vi "NE-500 FGV.vi"(7 "Function":T2(ring), 8 "error in":errorcluster, 10 "Setting":T1, 11 "VISA resource":refnum<visa-resource-name>) -> (0 "error out":errorcluster, 3 "Read String":string)   [LabVIEW 2019, in "NE-500.lvlib"]
uses:
  NE-500.lvlib
  <vilib>/Instr/_visa.llb/VISA Configure Serial Port (Instr).vi
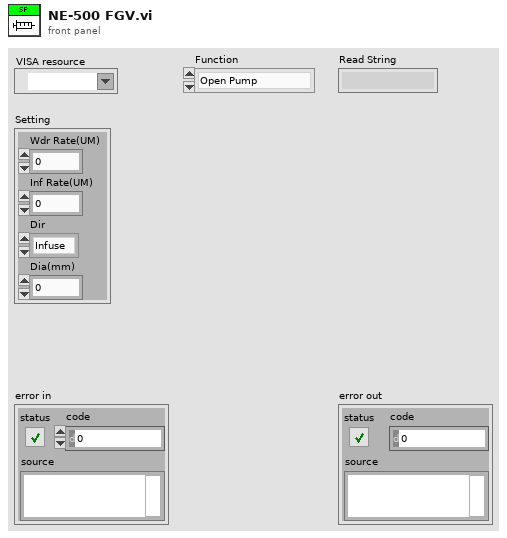
[diagram p1: front panel]
types:
  T1 = cluster{"Wdr Rate(UM)":dbl, "Inf Rate(UM)":dbl, "Dir":enum16{"Infuse", "Withdraw"}, "Dia(mm)":dbl}
  T2 = enum16{"Open Pump", "Read", "Set", "Run", "Stop", "Close Pump"}
  T3 = cluster{"Syringe Pump Setting":cluster{"Wdr Rate(UM)":dbl, "Inf Rate(UM)":dbl, "Dir":enum16{"Infuse", "Withdraw"}, "Dia(mm)":dbl}, "On/Off":bool, "VISA resource":refnum<visa-resource-name>, "Read String":string}
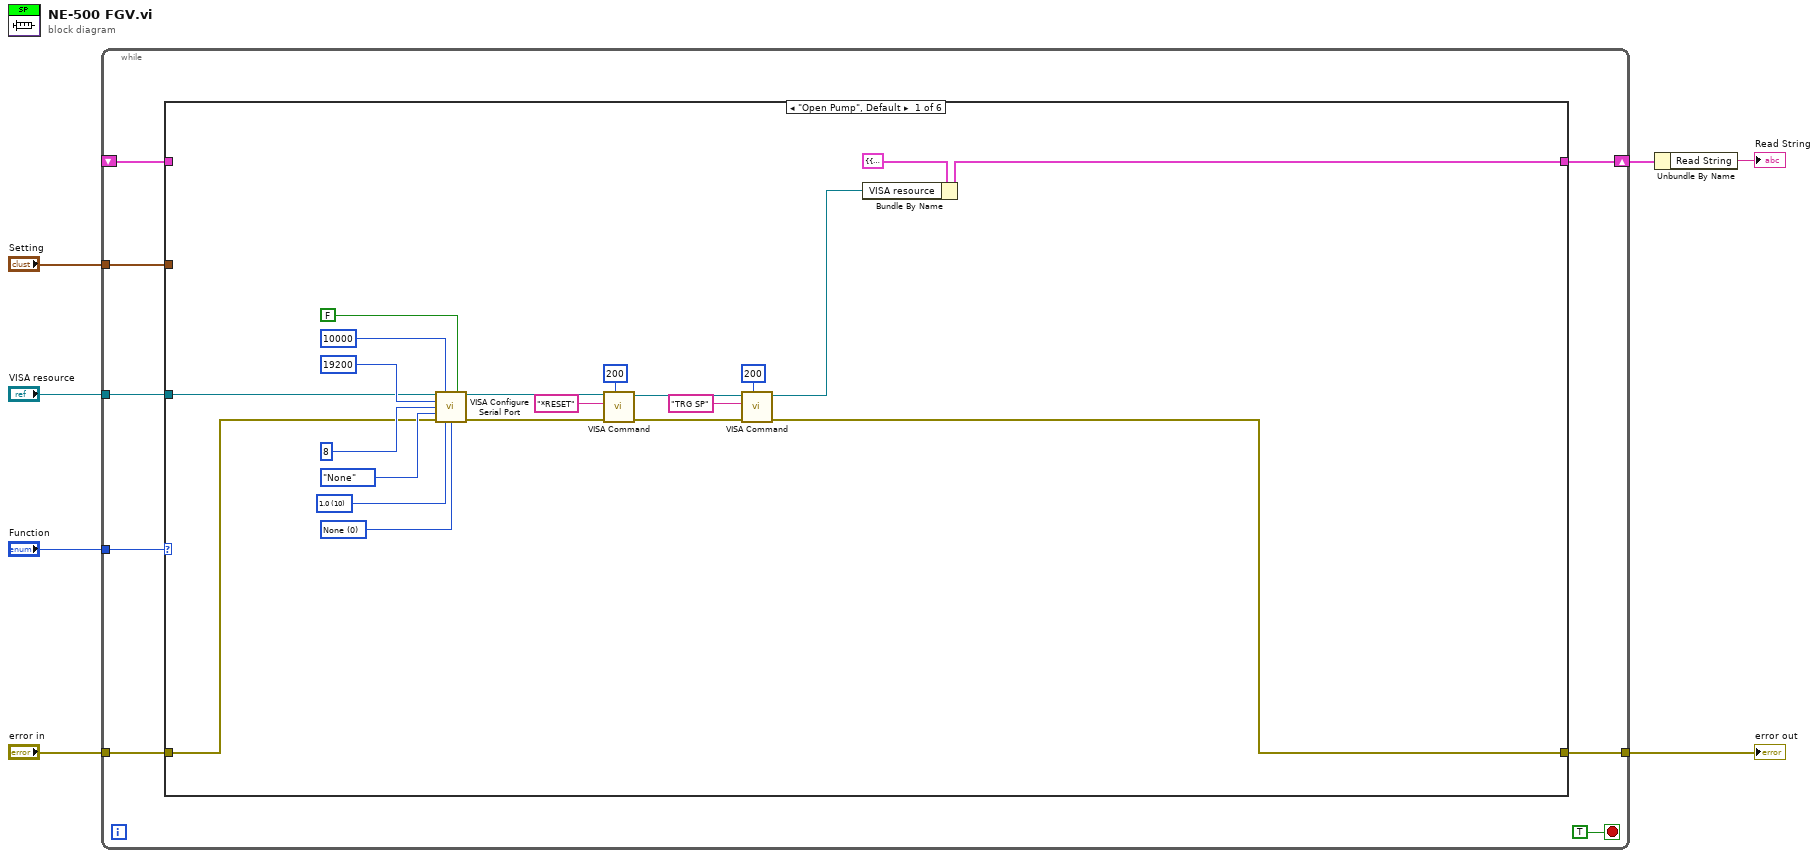
[diagram p0: block diagram]
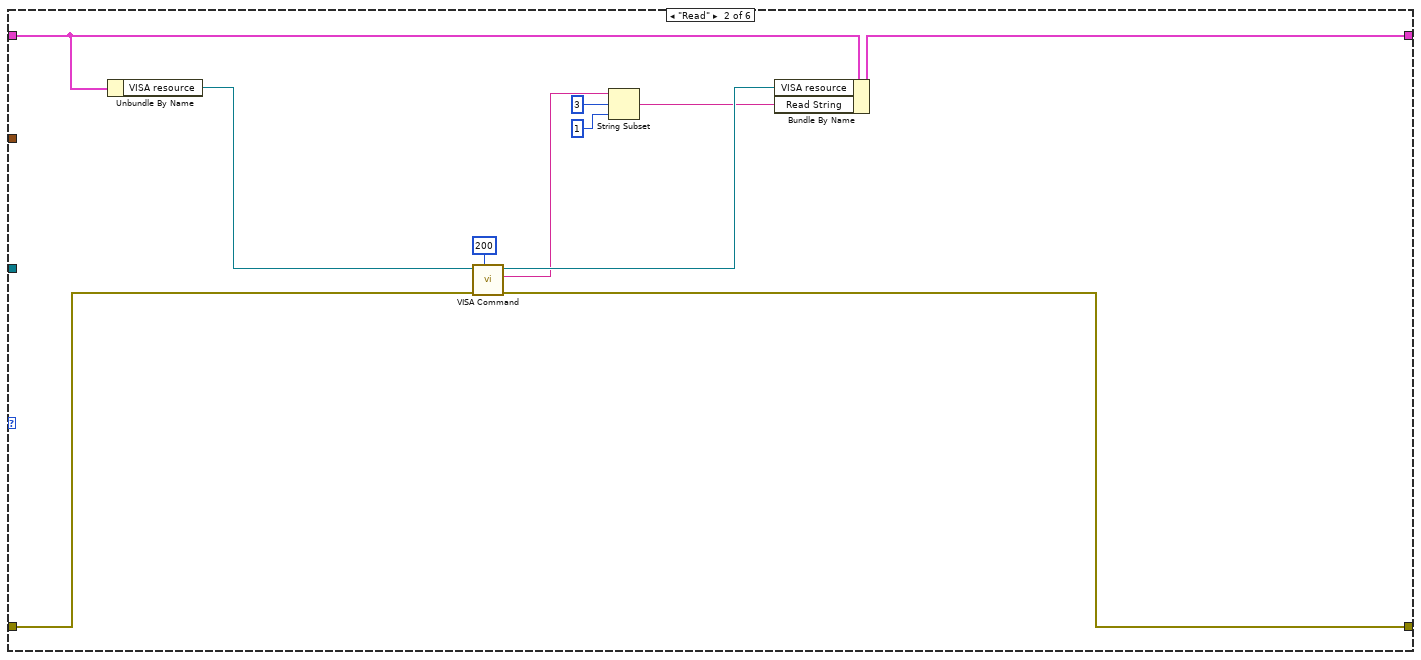
[diagram p2: hidden frame]
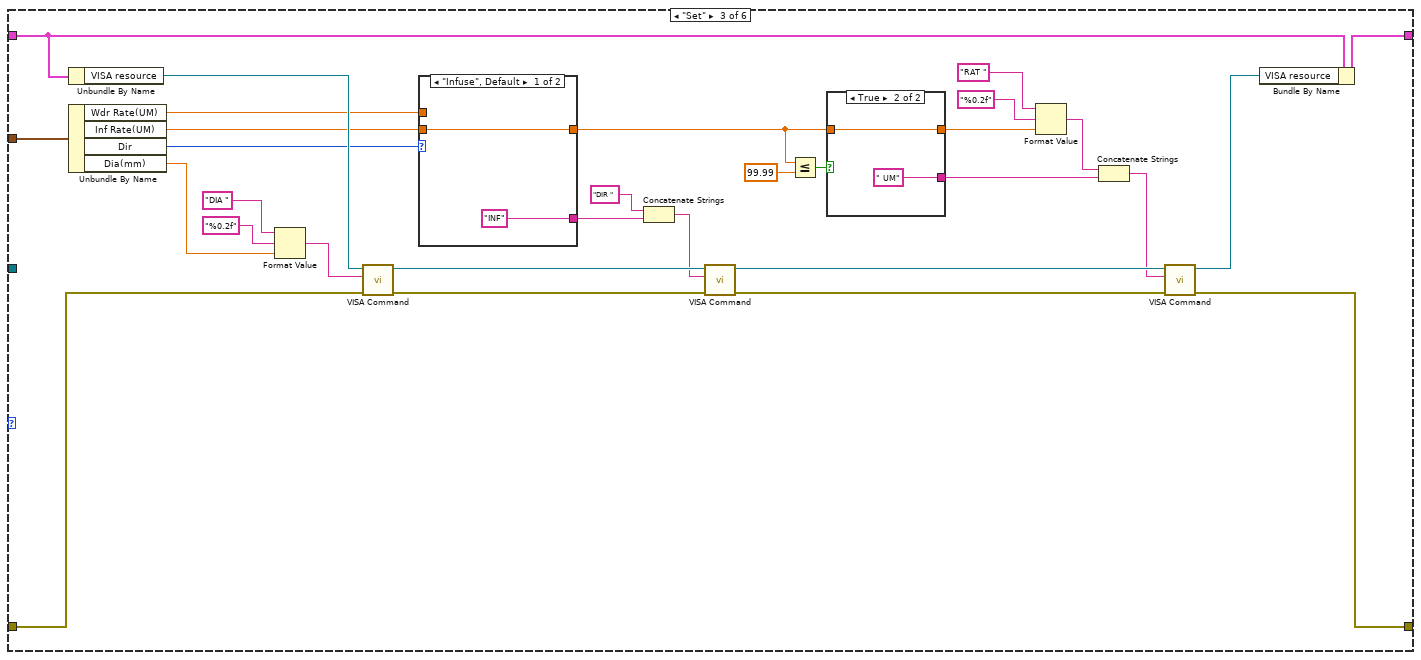
[diagram p3: hidden frame]
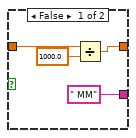
[diagram p4: hidden frame]
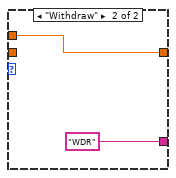
[diagram p5: hidden frame]
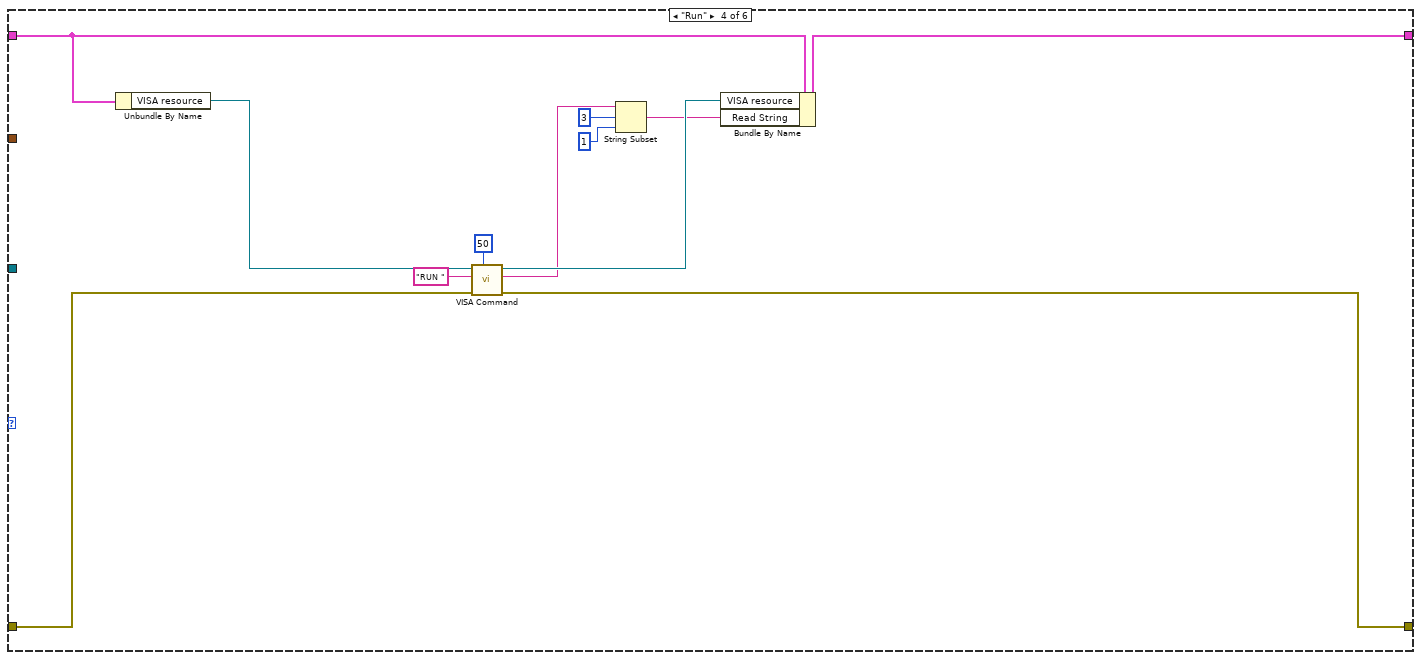
[diagram p6: hidden frame]
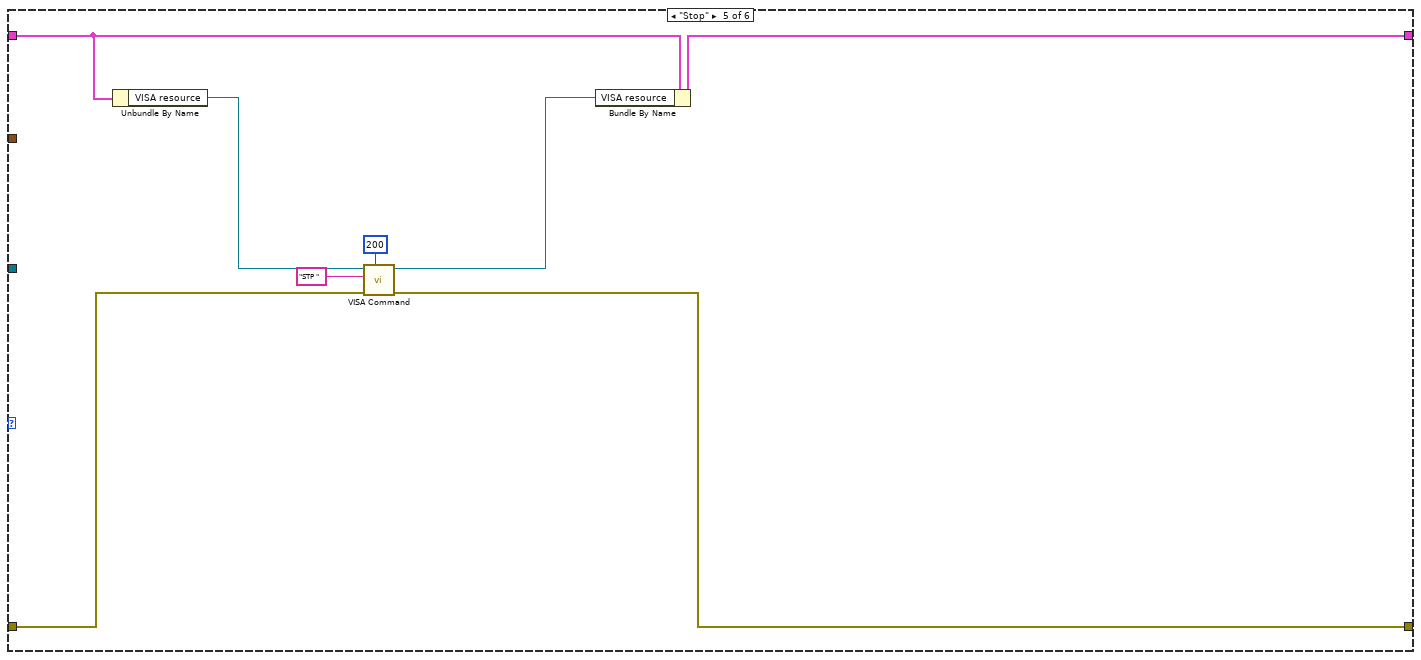
[diagram p7: hidden frame]
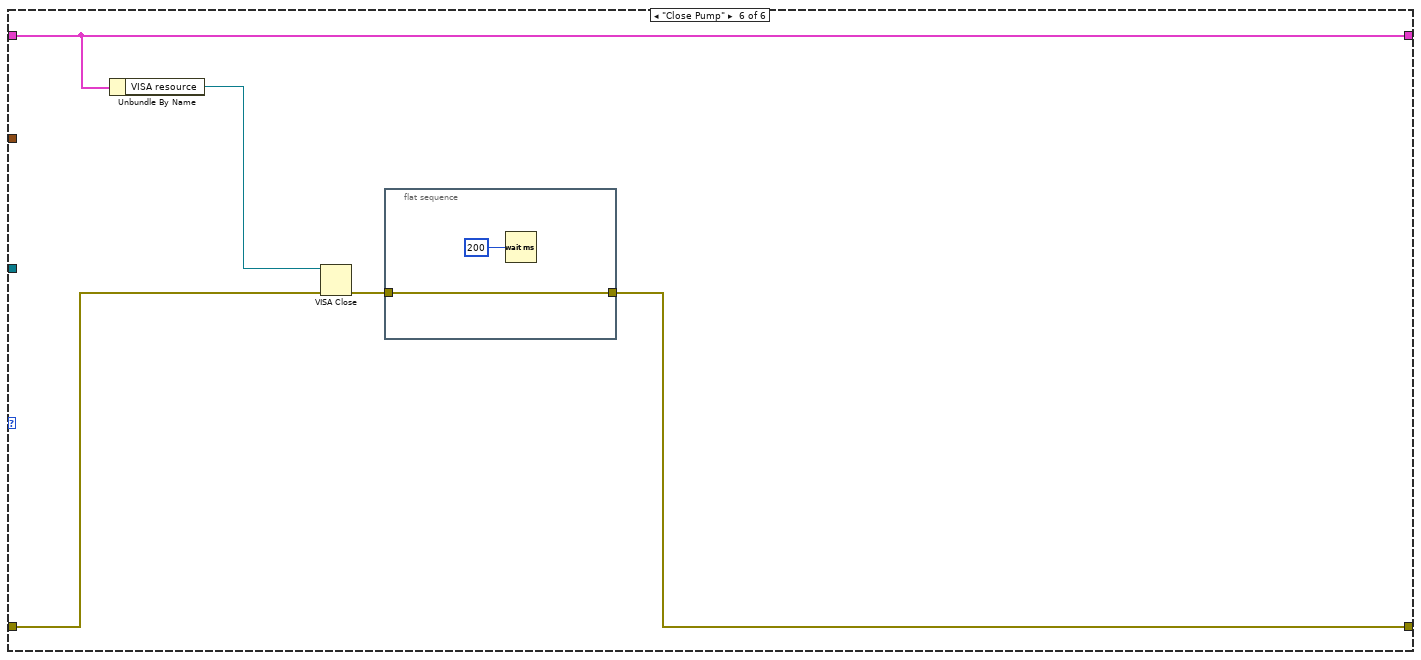
[diagram p8: hidden frame]
diagram:
  n1 = while {
    tunnel: "Function" -> [w14]
    shift-right: [w12] -> w2
    shift-left: _ -> [w13]
    tunnel: "VISA resource" -> [w11]
    tunnel: "error in" -> [w10]
    tunnel: [w9] -> w4
    tunnel: "Setting" -> [w8]
    stop <- TRUE stop-if-true
    n2 = case shown="\"Open Pump\", Default" w14 {
      tunnel: w13 -> [_ w45 w65 w97 w105 w111]
      tunnel: [w27 w44 w57 w93 w101 w111] -> w12
      tunnel: w11 -> [w28 _ _ _ _ _]
      tunnel: w10 -> [w29 w47 w71 w99 w107 w112]
      tunnel: [w18 w46 w68 w98 w102 w108] -> w9
      tunnel: w8 -> [_ _ w67 _ _ _]
      frame "Open Pump", Default {
        w33 = u16 0 items=["None"=0, "XON/XOFF"=1, "RTS/CTS"=2, "DTR/DSR"=4] ("flow control")
        w32 = u16 10 items=["1.0"=10, "1.5"=15, "2.0"=20] ("stop bits")
        n3 = call-poly "VISA Configure Serial Port"("VISA resource name"=w28, "timeout (10sec)"=u32 10000, "Enable Termination\nChar (T)"=FALSE ("Enable Termination Char (T)"), "baud rate (9600)"=u32 19200 ("baud rate"), "data bits (8)"=u16 8 ("data bits"), "parity (0:none)"=enum16{"None", "Odd", "Even", "Mark", "Space"}."None", "error in (no error)"=w29, "stop bits (10: 1 bit)"=w32, "flow control (0:none)"=w33) -> ("VISA resource name out"=w25:refnum<visa-resource-name>, "error out"=w26:errorcluster)  [unwired: 5 out]
        n4 = call "VISA Command.vi"("Wait (ms)"=u32 200, "error in (no error)"=w26, "Command"="*RESET" ("CMD string"), "VISA resource name"=w25) -> ("error out"=w24:errorcluster, "VISA resource name out"=w21:refnum<visa-resource-name>)  [unwired: 5 in, 1 out]
        n5 = call "VISA Command.vi"("Wait (ms)"=u32 200, "error in (no error)"=w24, "Command"="TRG SP" ("CMD string"), "VISA resource name"=w21) -> ("error out"=w18:errorcluster, "VISA resource name out"=w17:refnum<visa-resource-name>)  [unwired: 5 in, 1 out]
        n6 = Bundle By Name(cluster=T3 {"Syringe Pump Setting"={"Wdr Rate(UM)"=0.0, "Inf Rate(UM)"=0.0, "Dir"=enum."Infuse", "Dia(mm)"=0.0}, "On/Off"=FALSE, "VISA resource"="", "Read String"=""}, "VISA resource"=w17) -> (w27:T3)
      }
      frame "Read" {
        n7 = Unbundle By Name(w45) -> ("VISA resource"=w43:refnum<visa-resource-name>)
        n8 = call "VISA Command.vi"("Wait (ms)"=u32 200, "error in (no error)"=w47, "VISA resource name"=w43) -> ("error out"=w46:errorcluster, "read buffer"=w38:string, "VISA resource name out"=w42:refnum<visa-resource-name>)  [unwired: 6 in]
        n9 = String Subset(string=w38, offset (0)=3, length (rest)=1 ("length (rest)")) -> (substring=w37:string)
        n10 = Bundle By Name(cluster=w45, "VISA resource"=w42, "Read String"=w37) -> (w44:T3)
      }
      frame "Set" {
        n11 = Unbundle By Name(w65) -> ("VISA resource"=w64:refnum<visa-resource-name>)
        n12 = Unbundle By Name(w67) -> ("Wdr Rate(UM)"=w61:dbl, "Inf Rate(UM)"=w60:dbl, "Dir"=w62:enum16{"Infuse", "Withdraw"}, "Dia(mm)"=w63:dbl)
        n13 = Format Value(string ("")="DIA ", format string="%0.2f", value (0)=w63) -> (output string=w66:string)
        n14 = call "VISA Command.vi"("error in (no error)"=w71, "Command"=w66, "VISA resource name"=w64) -> ("error out"=w70:errorcluster, "VISA resource name out"=w59:refnum<visa-resource-name>)  [unwired: 6 in, 1 out]
        n15 = case shown="\"Infuse\", Default" w62 {
          tunnel: w61 -> [_ w86]
          tunnel: w60 -> [w84 _]
          tunnel: ["INF" "WDR"] -> w55
          tunnel: [w84 w86] -> w51
          frame "Infuse", Default {
          }
          frame "Withdraw" {
          }
        }
        n16 = Concatenate Strings("DIR " ("string"), w55) -> (w54:string)
        n17 = call "VISA Command.vi"("error in (no error)"=w70, "Command"=w54, "VISA resource name"=w59) -> ("error out"=w69:errorcluster, "VISA resource name out"=w58:refnum<visa-resource-name>)  [unwired: 6 in, 1 out]
        n18 = Less Or Equal?(x=w51, y=99.99) -> (x <= y?=w52:bool)
        n19 = case shown="True" w52 {
          tunnel: w51 -> [w81 w83]
          tunnel: [w80 w83] -> w50
          tunnel: [" MM" " UM"] -> w49
          frame False {
            n20 = Divide(x=w81, y=1000.0) -> (x/y=w80:dbl)
          }
          frame True {
          }
        }
        n21 = Format Value(string ("")="RAT ", format string="%0.2f", value (0)=w50) -> (output string=w74:string)
        n22 = Concatenate Strings(w74, w49) -> (w48:string)
        n23 = call "VISA Command.vi"("error in (no error)"=w69, "Command"=w48, "VISA resource name"=w58) -> ("error out"=w68:errorcluster, "VISA resource name out"=w56:refnum<visa-resource-name>)  [unwired: 6 in, 1 out]
        n24 = Bundle By Name(cluster=w65, "VISA resource"=w56) -> (w57:T3)
      }
      frame "Run" {
        n25 = Unbundle By Name(w97) -> ("VISA resource"=w95:refnum<visa-resource-name>)
        n26 = call "VISA Command.vi"("Wait (ms)"=u32 50, "error in (no error)"=w99, "Command"="RUN " ("string (\"\")"), "VISA resource name"=w95) -> ("error out"=w98:errorcluster, "read buffer"=w89:string, "VISA resource name out"=w92:refnum<visa-resource-name>)  [unwired: 5 in]
        n27 = String Subset(string=w89, offset (0)=3, length (rest)=1 ("length (rest)")) -> (substring=w88:string)
        n28 = Bundle By Name(cluster=w97, "VISA resource"=w92, "Read String"=w88) -> (w93:T3)
      }
      frame "Stop" {
        n29 = Unbundle By Name(w105) -> ("VISA resource"=w104:refnum<visa-resource-name>)
        n30 = call "VISA Command.vi"("Wait (ms)"=u32 200, "error in (no error)"=w107, "Command"="STP " ("string (\"\")"), "VISA resource name"=w104) -> ("error out"=w102:errorcluster, "VISA resource name out"=w100:refnum<visa-resource-name>)  [unwired: 5 in, 1 out]
        n31 = Bundle By Name(cluster=w105, "VISA resource"=w100) -> (w101:T3)
      }
      frame "Close Pump" {
        n32 = Unbundle By Name(w111) -> ("VISA resource"=w110:refnum<visa-resource-name>)
        n33 = VISA Close(VISA resource name=w110, error in (no error)=w112) -> (error out=w109:errorcluster)
        n34 = flat-sequence {
          tunnel: w109 -> [w114]
          tunnel: [w114] -> w108
          frame #0 {
            n35 = Wait (ms)(milliseconds to wait=u32 200) -> ()  [unwired: 1 out]
          }
        }
      }
    }
  }
  "error out" <- w4
  n36 = Unbundle By Name(w2) -> ("Read String"=→"Read String":string)
